vi "Write to COM Port.vi"(8 "error in":errorcluster caption="error IO", 10 "Command (input)":string, 11 "VISA resource name in":refnum<visa-resource-name>) -> (0 "error out":errorcluster, 3 "VISA resource name out":refnum<visa-resource-name>)   [LabVIEW 2015, in "JULABO DeviceDriver.lvlib"]
uses:
  JULABO DeviceDriver.lvlib
panel:
  out "Command (Debug)":string
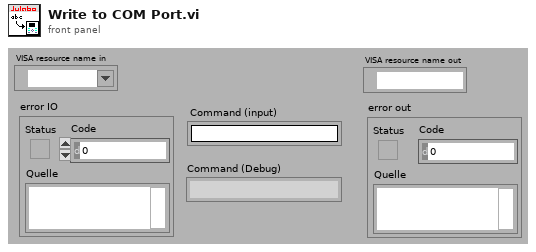
[diagram p1: front panel]
types:
  T1 = typedef "JULABO DeviceDriver.lvlib/InstrumentType.ctl" = enum8{"Default", "FC-Series", "HT30/HT60", "LC4"}
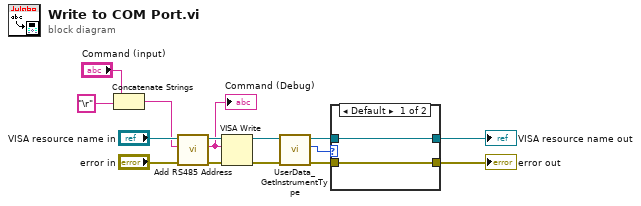
[diagram p0: block diagram]
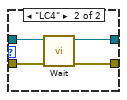
[diagram p2: hidden frame]
diagram:
  n1 = Concatenate Strings("Command (input)", "\r" ("String")) -> (w9:string)
  n2 = call "Add RS485 Address.vi"("error in"="error in", "Command (input)"=w9, "VISA resource name in"="VISA resource name in") -> ("error out"=w13:errorcluster, "Command (output)"=w11:string, "VISA resource name out"=w12:refnum<visa-resource-name>)  [unwired: 2 in]
  "Command (Debug)" <- w11
  n3 = VISA Write(VISA resource name=w12, write buffer=w11, error in (no error)=w13) -> (VISA resource name out=w5:refnum<visa-resource-name>, error out=w4:errorcluster)  [unwired: 1 out]
  n4 = call "UserData_GetInstrumentType.vi"("Fehler (Eingang)"=w4, "VISA resource name in"=w5) -> ("Fehler (Ausgang)"=w6:errorcluster, "InstrumentType"=w3:T1, "VISA resource name out"=w7:refnum<visa-resource-name>)  [unwired: 3 in]
  n5 = case shown="Default" w3 {
    tunnel: w7 -> [w17 w21]
    tunnel: w6 -> [w16 w20]
    tunnel: [w17 w19] -> w2
    tunnel: [w16 w18] -> w1
    frame Default {
    }
    frame "LC4" {
      n6 = call "Wait.vi"("error in"=w20, "VISA resource name in"=w21) -> ("error out"=w18:errorcluster, "VISA resource name out"=w19:refnum<visa-resource-name>)  [unwired: 4 in]
    }
  }
  "error out" <- w1
  "VISA resource name out" <- w2
